vi "CSC_GetBodies.vi"(8 "error in (no error)":errorcluster, 11 "CableSerialChain in":refnum<class "CableSerialChain.lvclass">) -> (0 "error out":errorcluster, 2 "Bodies":refnum<class "Bodies.lvclass">, 3 "CableSerialChain out":refnum<class "CableSerialChain.lvclass">)   [LabVIEW 2014, in "CableSerialChain.lvclass"]
uses:
  CableSerialChain.lvclass
  Body/Bodies.lvclass
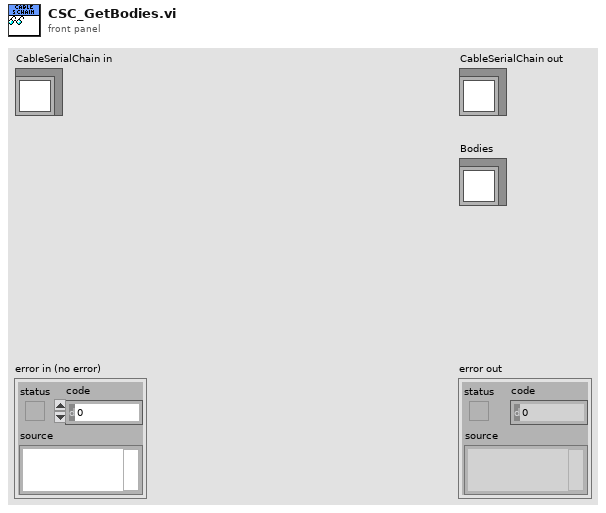
[diagram p1: front panel]
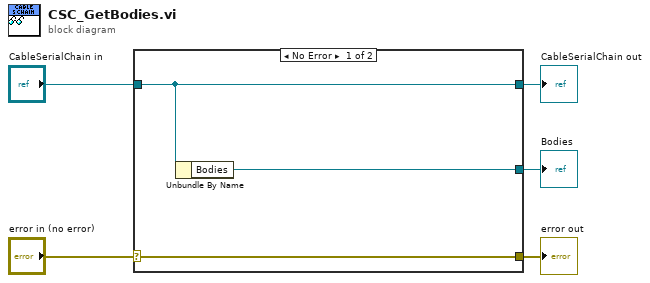
[diagram p0: block diagram]
diagram:
  n1 = case shown="No Error" "error in (no error)" {
    selector: "error in (no error)" -> [w8 w9]
    tunnel: [w8 w9] -> w4
    tunnel: [w7 w10] -> w2
    tunnel: "CableSerialChain in" -> [w7 w10]
    tunnel: [w6 _] -> w1
    frame No Error {
      n2 = Unbundle By Name(w7) -> ("Bodies"=w6:refnum<class "Bodies.lvclass">)
    }
    frame Error {
    }
  }
  "error out" <- w4
  "CableSerialChain out" <- w2
  "Bodies" <- w1
